vi "Measurement Init.vi"(8 "error in (no error)":errorcluster, 9 "Measurement Names":string[](array[string]), 10 "Table description":T1={"ActiveCell"={"Row"=-2, "Column"=-2}, "CellBGColor"=0, "CellFontSize"=20, "CellFontBold"=TRUE, "CellFontColor"=0, "CellJustification"=enum."Center", "CellWidth"=122, "NumberOfRows"=0, "AutosizingRowHeight"=TRUE, "SizeHeight"=105, "Position"={"Left"=0, "Top"=0}, "TableWidth"=0, "RowHeaderHeight"=0, "RowHeaderColor"=0}, 11 "ZenGage v3.0 UI in":refnum<class "ZenGage v3.0 UI.lvclass">) -> (0 "error out":errorcluster, 3 "ZenGage v3.0 UI out":refnum<class "ZenGage v3.0 UI.lvclass">)   [LabVIEW 2015, in "ZenGage v3.0 UI.lvclass"]
uses:
  ZenGage v3.0 UI.lvclass
  Type Definitions/Inspection/Table description.ctl
  <vilib>/Utility/miscctls.llb/LVRowAndColumnTypeDef.ctl
  <vilib>/Utility/miscctls.llb/LVPositionTypeDef.ctl
  ZenGage v3.0 UI.lvclass/ZenGage v3.0 UI.ctl
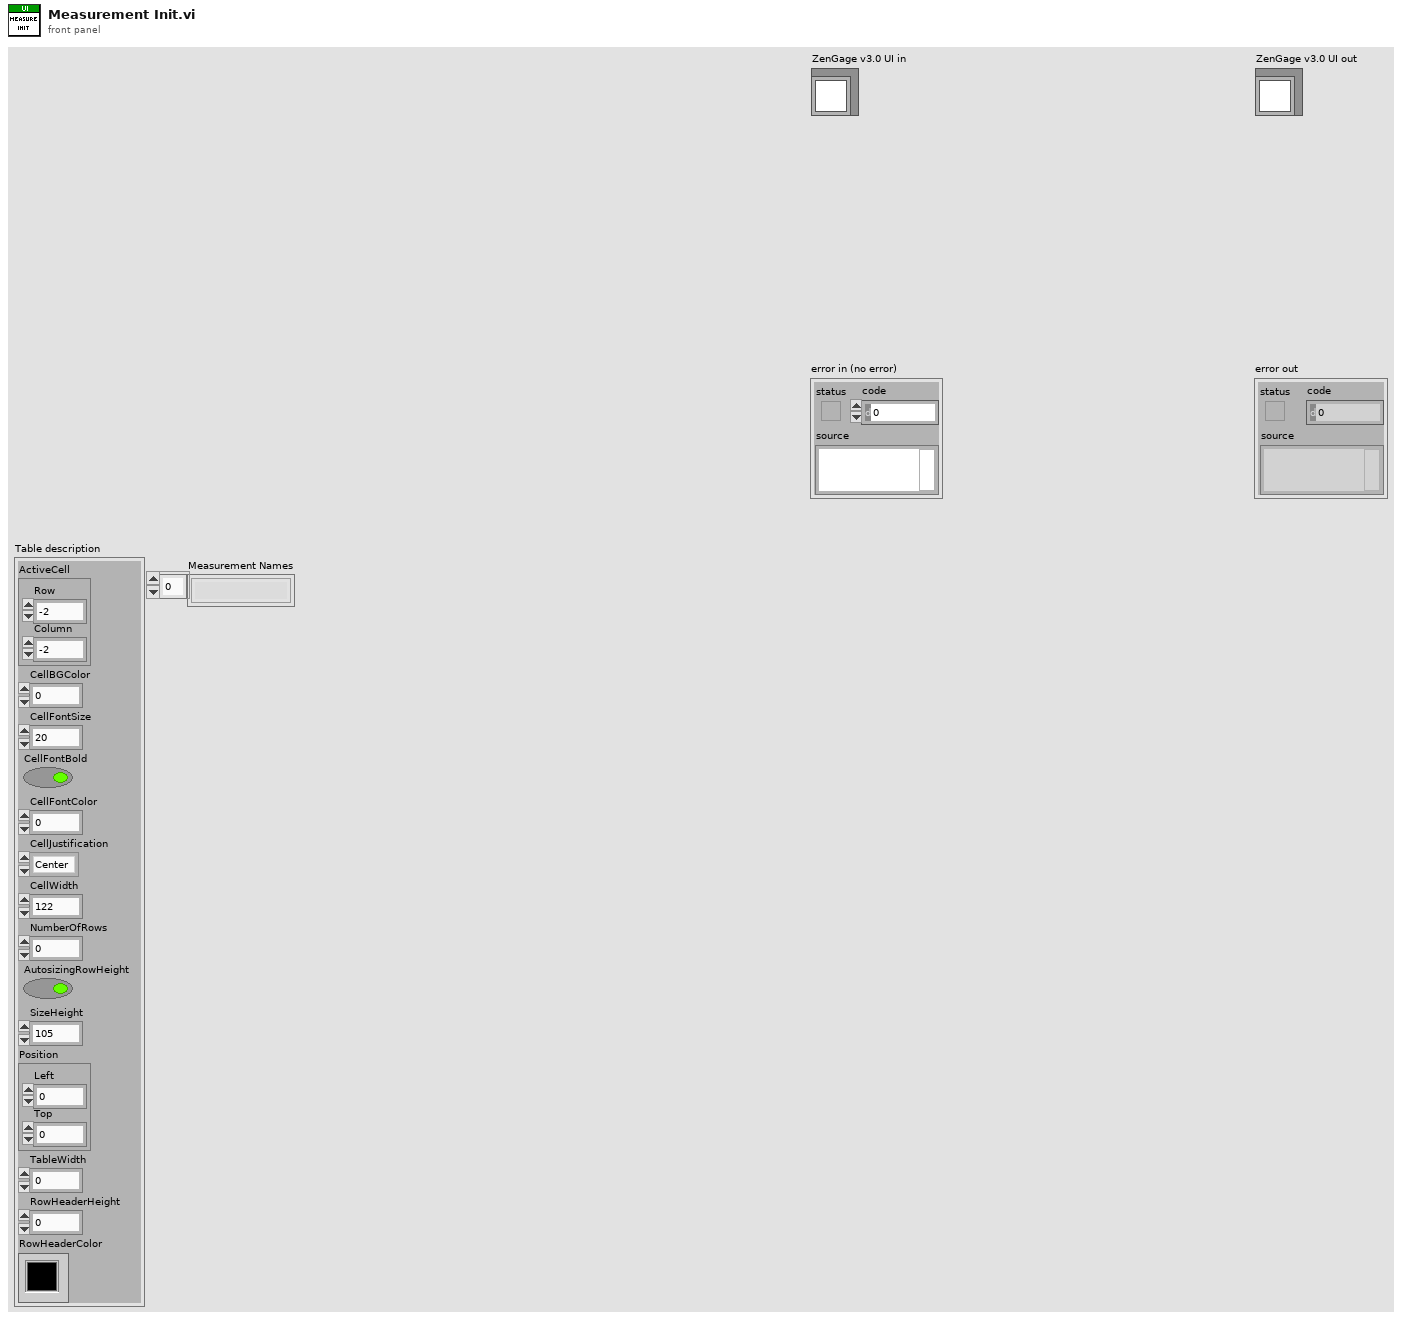
[diagram p1: front panel]
types:
  T1 = typedef "ZenGage v3.0 UI.lvclass/Table description.ctl" = cluster{"ActiveCell":T2, "CellBGColor":u32, "CellFontSize":u32, "CellFontBold":bool, "CellFontColor":u32, "CellJustification":enum16{"Left", "Center", "Right"}, "CellWidth":u32, "NumberOfRows":u32, "AutosizingRowHeight":bool, "SizeHeight":u32, "Position":T3, "TableWidth":u32, "RowHeaderHeight":u32, "RowHeaderColor":u32}
  T2 = typedef "LVRowAndColumnTypeDef.ctl" = cluster{"Row":i32, "Column":i32}
  T3 = typedef "LVPositionTypeDef.ctl" = cluster{"Left":i32, "Top":i32}
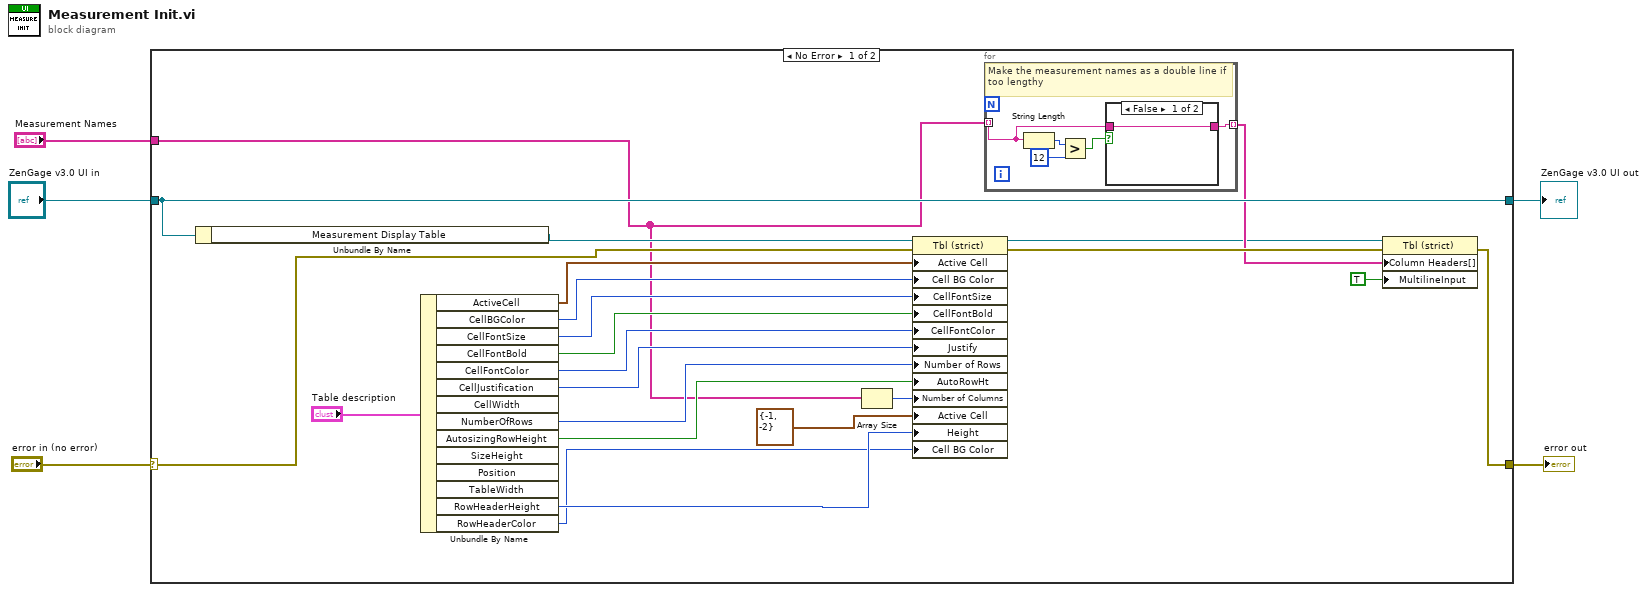
[diagram p0: block diagram]
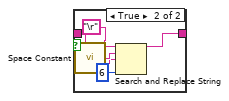
[diagram p2: hidden frame]
diagram:
  n1 = case shown="No Error" "error in (no error)" {
    selector: "error in (no error)" -> [w25 w40]
    tunnel: [w23 w40] -> w2
    tunnel: [w27 w39] -> w3
    tunnel: "ZenGage v3.0 UI in" -> [w27 w39]
    tunnel: "Measurement Names" -> [w6 _]
    frame No Error {
      n2 = Unbundle By Name(w27) -> ("Measurement Display Table"=w26:refnum<vi>)
      n3 = Unbundle By Name("Table description") -> ("ActiveCell"=w17:T2, "CellBGColor"=w16:u32, "CellFontSize"=w15:u32, "CellFontBold"=w14:bool, "CellFontColor"=w13:u32, "CellJustification"=w12:enum16{"Left", "Center", "Right"}, "NumberOfRows"=w11:u32, "AutosizingRowHeight"=w10:bool, "RowHeaderHeight"=w8:u32, "RowHeaderColor"=w7:u32)  [unwired: 4 out]
      n4 = Array Size(array=w6) -> (size(s)=w18:i32)
      n5 = property class="Tbl (strict)"(reference=w26, error in=w25, "Active Cell"=w17, "Cell BG Color"=w16, "CellFontSize"=w15, "CellFontBold"=w14, "CellFontColor"=w13, "Justify"=w12, "Number of Rows"=w11, "AutoRowHt"=w10, "Number of Columns"=w18, "Active Cell"=T2 {"Row"=-1, "Column"=-2} ("Active Cell:Active Cell"), "Height"=w8, "Cell BG Color"=w7) -> (reference out=w20:refnum<vi>, error out=w24:errorcluster)
      n6 = for {
        tunnel: w6 -> [w29] mode=indexing
        tunnel: [w28] -> w21 mode=indexing
        # "Make the measurement names as a double line if too lengthy"
        n7 = String Length(string=w29) -> (length=w32:i32)
        n8 = Greater?(x=w32, y=12) -> (0:w30:bool)
        n9 = case shown="False" w30 {
          tunnel: w29 -> [w33 w38]
          tunnel: [w33 w34] -> w28
          frame False {
          }
          frame True {
            n10 = call <vilib>:"Space Constant.vi"() -> ("String"=w37:string)
            n11 = Search and Replace String(input string=w38, search string=w37, replace string="\r", offset=6 ("offset (0)")) -> (result string=w34:string)  [unwired: 4 in, 3 out]
          }
        }
      }
      n12 = property class="Tbl (strict)"(reference=w20, error in=w24, "Column Headers[]"=w21, "MultilineInput"=TRUE ("Multiple Line Input")) -> (error out=w23:errorcluster)  [unwired: 1 out]
    }
    frame Error {
    }
  }
  "error out" <- w2
  "ZenGage v3.0 UI out" <- w3
